vi "CRYProject Tree Action Check.vi"(8 "tag":string, 9 "Coords In":T1={"Horizontal"=-1, "Vertical"=-1}, 10 "sOption":string, 11 "Project Tree reference":refnum<vi>) -> (2 "Type Out":string, 3 "bResult":bool)   [LabVIEW 2013]
uses:
  <vilib>/Utility/miscctls.llb/LVPoint32TypeDef.ctl
  CRYProject Editor Global.vi
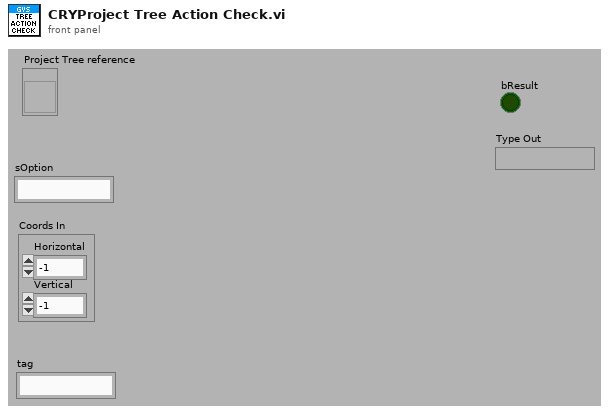
[diagram p1: front panel]
types:
  T1 = typedef "LVPoint32TypeDef.ctl" = cluster{"Horizontal":i32, "Vertical":i32}
  T2 = typedef "CRYTS.ctl" = cluster{"No.TS":u16, "TS File Path":path, "TS Name":string, "EditStepName":string, "Steps":T3[], "New State":bool, "Change State":bool, "Flattened CurveLib Data":string, "Document Data":string, "EditStepNo":u16, "Operator Start File":string, "Sequence Type":string, "Sequence Language":string}
  T3 = typedef "CRYStep.ctl" = cluster{"No.VI":i32, "Category":string, "StepName":string, "Seq setup flattened":string, "Comment":string, "Steps config.":bool[], "Jump config":i32[], "Start":dbl, "Increment":dbl, "Name":string, "Unit":string, "Y data":u16, "Y prefix":string, "Y dB ref":dbl, "Y unit":string, "Repeat State Array":cluster{"Start":dbl, "Increment":dbl, "Count":i32, "Num":i32}[]}
  T4 = enum16{"OK", "Yes", "YesNo", "YesNoCancel", "ReplaceAppend"}
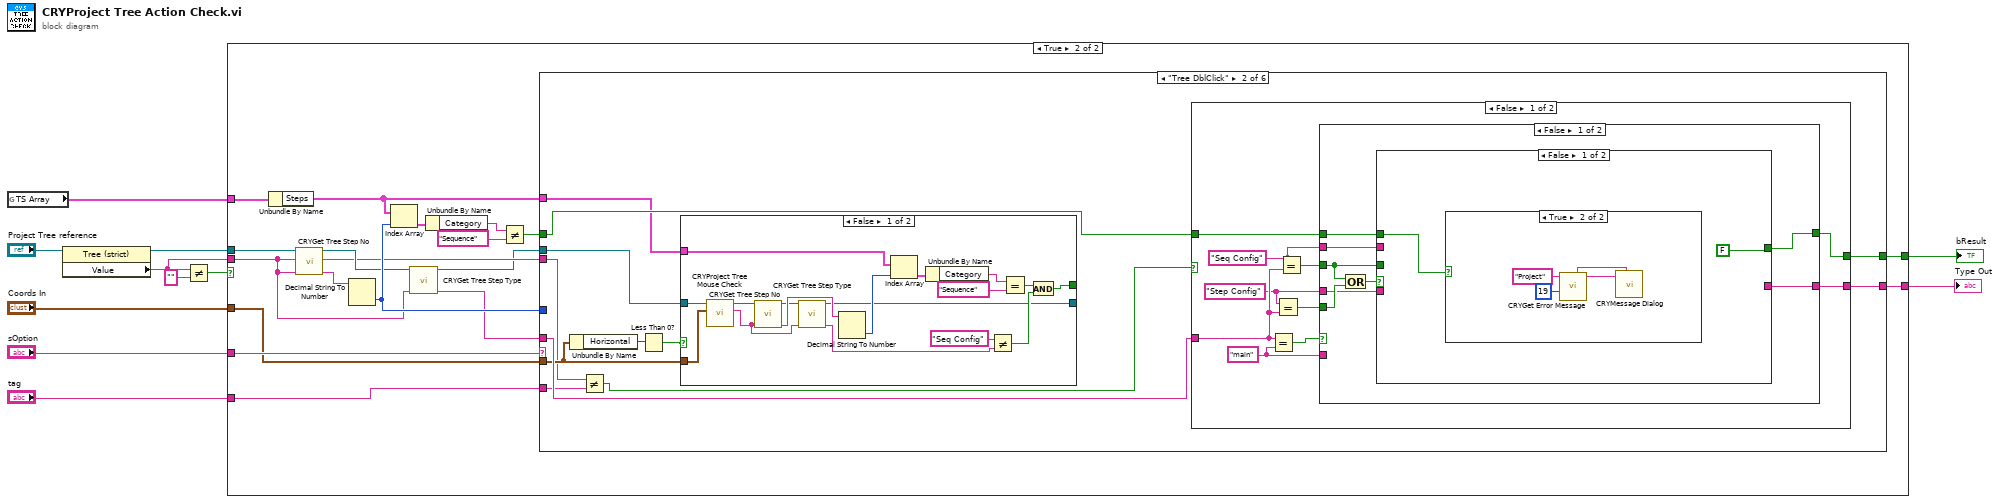
[diagram p0: block diagram]
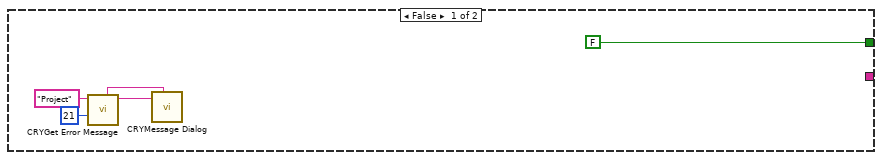
[diagram p2: hidden frame]
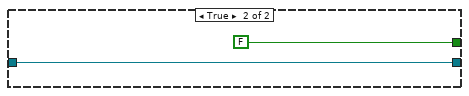
[diagram p4: hidden frame]
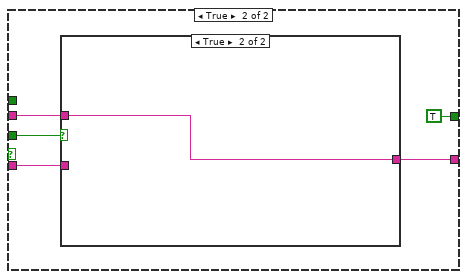
[diagram p6: hidden frame]
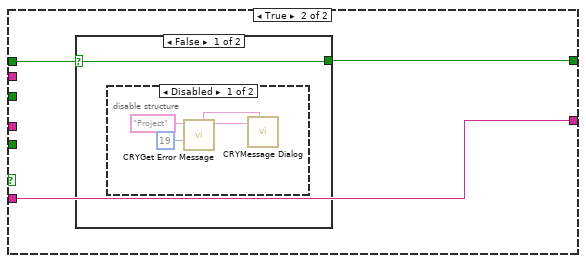
[diagram p8: hidden frame]
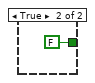
[diagram p11: hidden frame]
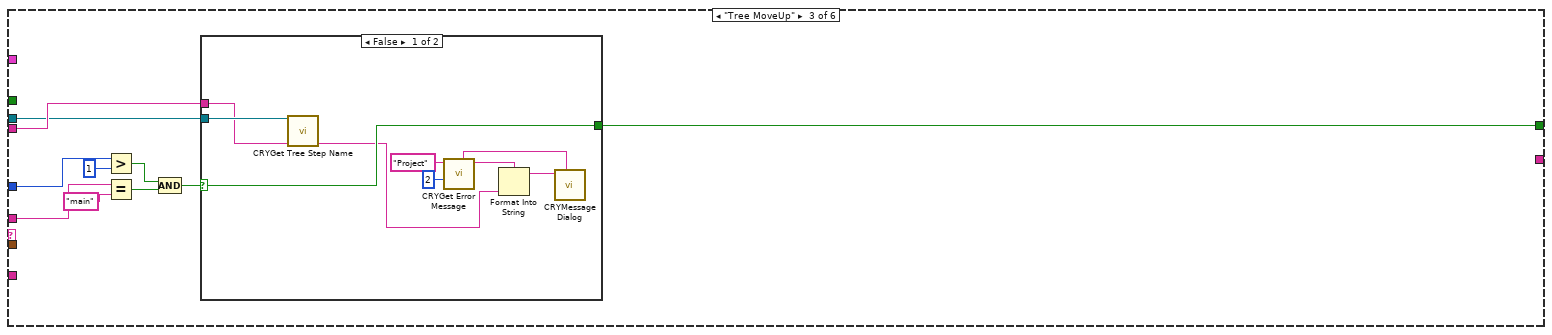
[diagram p12: hidden frame]
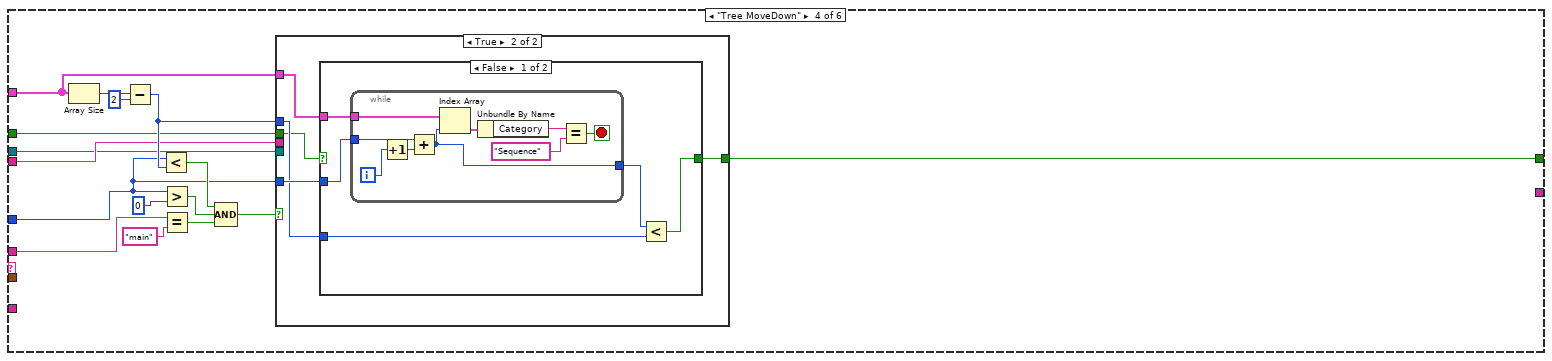
[diagram p14: hidden frame]
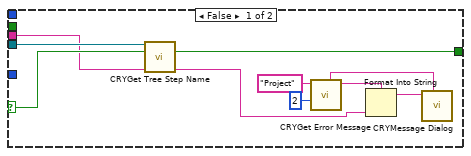
[diagram p15: hidden frame]
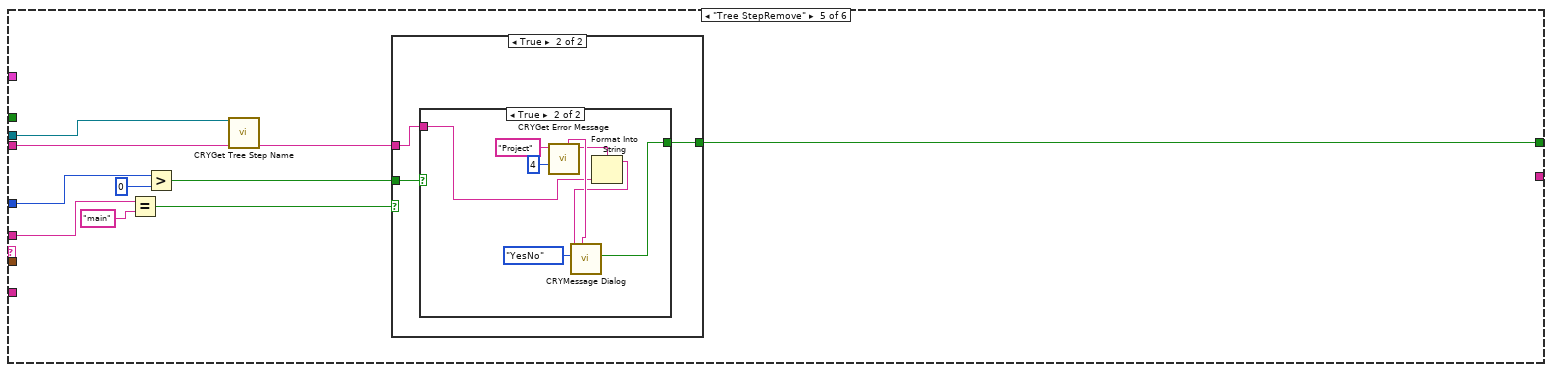
[diagram p17: hidden frame]
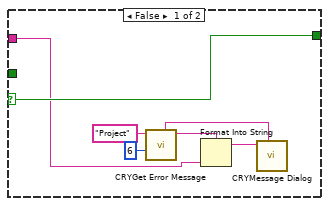
[diagram p18: hidden frame]
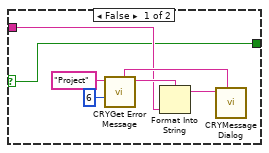
[diagram p19: hidden frame]
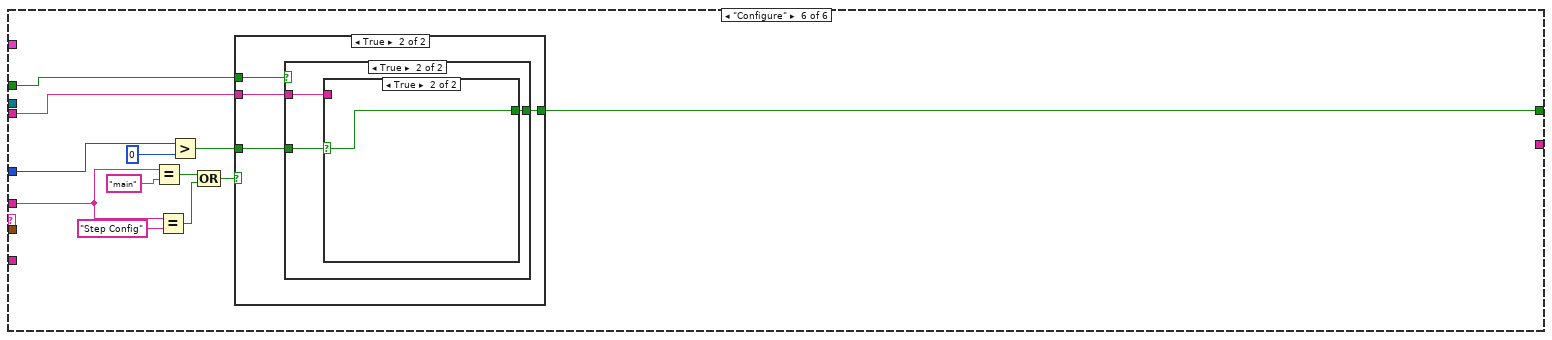
[diagram p20: hidden frame]
diagram:
  n1 = global read "CRYProject Editor Global.vi" "TS Array"() -> (w4:T2)
  n2 = property on="Property Node" class="Tree (strict)"(reference="Project Tree reference") -> (reference out=w8:refnum<vi>, "Value"=w2:string)  [unwired: 1 in, 1 out]
  n3 = Not Equal?(x=w2, y="") -> (x != y?=w7:bool)
  n4 = case shown="True" w7 {
    tunnel: [FALSE ("YesNo") w34] -> w11
    tunnel: "sOption" -> [_ w33]
    tunnel: w8 -> [_ w23]
    tunnel: w2 -> [_ w20]
    tunnel: "Coords In" -> [_ w24]
    tunnel: w4 -> [_ w31]
    tunnel: [_ w30] -> w3
    tunnel: "tag" -> [_ w17]
    frame False {
      n5 = call "CRYGet Error Message.vi"("Error No"=21, "Kind"="Project") -> ("Message"=w15:string, "Window Title"=w14:string)  [unwired: 4 in, 4 out]
      n6 = call "CRYMessage Dialog.vi"("Window Title"=w14, "Message Content"=w15) -> ()  [unwired: 8 in, 2 out]
    }
    frame True {
      n7 = Unbundle By Name(w31) -> ("Steps"=w32:T3[])
      n8 = call "CRYGet Tree Step No.vi"("SequenceTree"=w23, "Active Item Tag"=w20) -> ("reference out"=w21:refnum<vi>, "Active Cell String4"=w22:string)  [unwired: 12 in]
      n9 = Decimal String To Number(string=w22) -> (number=w25:i32)  [unwired: 2 in, 1 out]
      n10 = Index Array(array=w32, index=w25) -> (element=w28:T3)
      n11 = call "CRYGet Tree Step Type.vi"("SequenceTree"=w21, "Active Item Tag"=w20) -> ("reference out"=w18:refnum<vi>, "Active Cell String3"=w19:string)  [unwired: 12 in]
      n12 = Unbundle By Name(w28) -> ("Category"=w29:string)
      n13 = Not Equal?(x=w29, y="Sequence" ("Category")) -> (x != y?=w26:bool)
      n14 = case shown="\"Tree DblClick\"" w33 {
        tunnel: w18 -> [_ w39 w108 w129 w174 _]
        tunnel: [_ w46 w116 w142 w181 w218] -> w34
        tunnel: w32 -> [_ w38 _ w138 _ _]
        tunnel: w20 -> [_ w36 w111 w132 w173 w214]
        tunnel: w19 -> [_ w44 w110 w131 w177 w208]
        tunnel: w26 -> [_ w45 _ w128 _ w213]
        tunnel: w25 -> [_ _ w109 w130 w176 w212]
        tunnel: [_ w43 _ _ _ _] -> w30
        tunnel: w24 -> [_ w40 _ _ _ _]
        tunnel: w17 -> [_ w37 _ _ _ _]
        frame Default {
        }
        frame "Tree DblClick" {
          n15 = Unbundle By Name(w40) -> ("Horizontal"=w42:i32)
          n16 = Not Equal?(x=w36, y=w37) -> (x != y?=w35:bool)
          n17 = Less Than 0?(x=w42) -> (x < 0?=w41:bool)
          n18 = case shown="False" w41 {
            tunnel: w39 -> [w63 w65]
            tunnel: w40 -> [w62 _]
            tunnel: [w48 w65] -> _
            tunnel: w38 -> [w57 _]
            tunnel: [w55 FALSE] -> _
            frame False {
              n19 = call "CRYProject Tree Mouse Check.vi"("Coords In"=w62, "Tree Reference In"=w63) -> ("Clicked String Out"=w49:string, "Tree Reference Out"=w52:refnum<vi>)  [unwired: 8 in]
              n20 = call "CRYGet Tree Step No.vi"("SequenceTree"=w52, "Active Item Tag"=w49) -> ("reference out"=w50:refnum<vi>, "Active Cell String4"=w51:string)  [unwired: 12 in]
              n21 = call "CRYGet Tree Step Type.vi"("SequenceTree"=w50, "Active Item Tag"=w49) -> ("reference out"=w48:refnum<vi>, "Active Cell String3"=w47:string)  [unwired: 12 in]
              n22 = Decimal String To Number(string=w51) -> (number=w58:i32)  [unwired: 2 in, 1 out]
              n23 = Index Array(array=w57, index=w58) -> (element=w60:T3)
              n24 = Unbundle By Name(w60) -> ("Category"=w59:string)
              n25 = Not Equal?(x="Seq Config" ("SequenceName"), y=w47) -> (x != y?=w53:bool)
              n26 = Equal?(x=w59, y="Sequence" ("Category")) -> (x = y?=w56:bool)
              n27 = Compound Arithmetic op=AND(w56, w53) -> (w55:bool)
            }
            frame True {
            }
          }
          n28 = case shown="False" w35 {
            tunnel: [w75 FALSE] -> w46
            tunnel: w45 -> [w73 _]
            tunnel: w44 -> [w72 _]
            tunnel: [w67 _] -> w43
            frame False {
              w68 = "Step Config" ("SequenceName")
              w69 = "Seq Config" ("SequenceName")
              w66 = "main" ("decimal integer string")
              n29 = Equal?(x=w72, y=w66) -> (x = y?=w74:bool)
              n30 = Equal?(x=w68, y=w72) -> (x = y?=w70:bool)
              n31 = Equal?(x=w69, y=w72) -> (x = y?=w71:bool)
              n32 = case shown="False" w74 {
                tunnel: w73 -> [w83 w99]
                tunnel: [w79 w98] -> w75
                tunnel: w71 -> [w80 _]
                tunnel: w70 -> [w82 _]
                tunnel: w69 -> [w78 _]
                tunnel: w68 -> [w77 _]
                tunnel: [w76 w97] -> w67
                tunnel: w66 -> [_ w97]
                frame False {
                  n33 = Compound Arithmetic op=OR(w80, w82) -> (w81:bool)
                  n34 = case shown="False" w81 {
                    tunnel: w83 -> [w85 _]
                    tunnel: w80 -> [_ w94]
                    tunnel: [FALSE TRUE] -> w79
                    tunnel: w78 -> [_ w92]
                    tunnel: w77 -> [_ w91]
                    tunnel: [_ w90] -> w76
                    frame False {
                      n35 = case shown="True" w85 {
                        frame False {
                        }
                        frame True {
                          n36 = call "CRYGet Error Message.vi"("Error No"=19, "Kind"="Project") -> ("Message"=w89:string, "Window Title"=w88:string)  [unwired: 4 in, 4 out]
                          n37 = call "CRYMessage Dialog.vi"("Window Title"=w88, "Message Content"=w89) -> ()  [unwired: 8 in, 2 out]
                        }
                      }
                    }
                    frame True {
                      n38 = case shown="True" w94 {
                        tunnel: w92 -> [_ w96]
                        tunnel: w91 -> [w95 _]
                        tunnel: [w95 w96] -> w90
                        frame False {
                        }
                        frame True {
                        }
                      }
                    }
                  }
                }
                frame True {
                  n39 = case shown="False" w99 {
                    selector: w99 -> [w100 w105]
                    tunnel: [w100 w105] -> w98
                    frame False {
                      n40 = disable-structure shown="Disabled" {
                        frame Disabled {
                          n41 = call "CRYGet Error Message.vi"("Error No"=19, "Kind"="Project") -> ("Message"=w104:string, "Window Title"=w103:string)  [unwired: 4 in, 4 out]
                          n42 = call "CRYMessage Dialog.vi"("Window Title"=w103, "Message Content"=w104) -> ()  [unwired: 8 in, 2 out]
                        }
                        frame Enabled {
                        }
                      }
                    }
                    frame True {
                    }
                  }
                }
              }
            }
            frame True {
            }
          }
        }
        frame "Tree MoveUp" {
          n43 = Greater?(x=w109, y=1) -> (0:w112:bool)
          n44 = Equal?(x=w110, y="main" ("decimal integer string")) -> (x = y?=w115:bool)
          n45 = Compound Arithmetic op=AND(w112, w115) -> (w114:bool)
          n46 = case shown="False" w114 {
            selector: w114 -> [w120 w126]
            tunnel: [w120 w126] -> w116
            tunnel: w108 -> [w119 _]
            tunnel: w111 -> [w118 _]
            frame False {
              n47 = call "CRYGet Tree Step Name.vi"("SequenceTree"=w119, "Active Item Tag"=w118) -> ("Active Cell String0"=w117:string)  [unwired: 12 in, 1 out]
              n48 = call "CRYGet Error Message.vi"("Error No"=2, "Kind"="Project") -> ("Message"=w123:string, "Window Title"=w125:string)  [unwired: 4 in, 4 out]
              n49 = Format Into String(format string=w123, w117) -> (resulting string=w124:string)  [unwired: 2 in, 1 out]
              n50 = call "CRYMessage Dialog.vi"("Window Title"=w125, "Message Content"=w124) -> ()  [unwired: 8 in, 2 out]
            }
            frame True {
            }
          }
        }
        frame "Tree MoveDown" {
          n51 = Array Size(array=w138) -> (size(s)=w141:i32)
          n52 = Subtract(x=w141, y=2) -> (x-y=w139:i32)
          n53 = Less?(x=w130, y=w139) -> (x < y?=w133:bool)
          n54 = Greater?(x=w130, y=0) -> (0:w135:bool)
          n55 = Equal?(x=w131, y="main" ("decimal integer string")) -> (x = y?=w137:bool)
          n56 = Compound Arithmetic op=AND(w133, w135, w137) -> (w136:bool)
          n57 = case shown="True" w136 {
            selector: w136 -> [w146 _]
            tunnel: [w146 w156] -> w142
            tunnel: w132 -> [w144 _]
            tunnel: w138 -> [_ w155]
            tunnel: w130 -> [_ w154]
            tunnel: w139 -> [_ w153]
            tunnel: w129 -> [w145 _]
            tunnel: w128 -> [_ w152]
            frame False {
              n58 = call "CRYGet Tree Step Name.vi"("SequenceTree"=w145, "Active Item Tag"=w144) -> ("Active Cell String0"=w143:string)  [unwired: 12 in, 1 out]
              n59 = call "CRYGet Error Message.vi"("Error No"=2, "Kind"="Project") -> ("Message"=w149:string, "Window Title"=w151:string)  [unwired: 4 in, 4 out]
              n60 = Format Into String(format string=w149, w143) -> (resulting string=w150:string)  [unwired: 2 in, 1 out]
              n61 = call "CRYMessage Dialog.vi"("Window Title"=w151, "Message Content"=w150) -> ()  [unwired: 8 in, 2 out]
            }
            frame True {
              n62 = case shown="False" w152 {
                selector: w152 -> [_ w171]
                tunnel: [w157 w171] -> w156
                tunnel: w155 -> [w161 _]
                tunnel: w154 -> [w160 _]
                tunnel: w153 -> [w158 _]
                frame False {
                  n63 = while {
                    tunnel: w161 -> [w170]
                    tunnel: w160 -> [w169]
                    tunnel: [w162] -> w159
                    i -> [w163]
                    stop <- w164 stop-if-true
                    n64 = Increment(x=w163) -> (x+1=w168:i32)
                    n65 = Add(x=w169, y=w168) -> (x+y=w162:i32)
                    n66 = Index Array(array=w170, index=w162) -> (element=w167:T3)
                    n67 = Unbundle By Name(w167) -> ("Category"=w166:string)
                    n68 = Equal?(x=w166, y="Sequence") -> (x = y?=w164:bool)
                  }
                  n69 = Less?(x=w159, y=w158) -> (x < y?=w157:bool)
                }
                frame True {
                }
              }
            }
          }
        }
        frame "Tree StepRemove" {
          n70 = Equal?(x=w177, y="main" ("decimal integer string")) -> (x = y?=w180:bool)
          n71 = Greater?(x=w176, y=0) -> (0:w178:bool)
          n72 = call "CRYGet Tree Step Name.vi"("SequenceTree"=w174, "Active Item Tag"=w173) -> ("Active Cell String0"=w172:string)  [unwired: 12 in, 1 out]
          n73 = case shown="True" w180 {
            selector: w180 -> [w188 _]
            tunnel: [w188 w191] -> w181
            tunnel: w172 -> [w182 w190]
            tunnel: w178 -> [_ w189]
            frame False {
              n74 = call "CRYGet Error Message.vi"("Error No"=6, "Kind"="Project") -> ("Message"=w185:string, "Window Title"=w187:string)  [unwired: 4 in, 4 out]
              n75 = Format Into String(format string=w185, w182) -> (resulting string=w186:string)  [unwired: 2 in, 1 out]
              n76 = call "CRYMessage Dialog.vi"("Window Title"=w187, "Message Content"=w186) -> ()  [unwired: 8 in, 2 out]
            }
            frame True {
              n77 = case shown="True" w189 {
                selector: w189 -> [w192 _]
                tunnel: [w192 w200] -> w191
                tunnel: w190 -> [w193 w199]
                frame False {
                  n78 = call "CRYGet Error Message.vi"("Error No"=6, "Kind"="Project") -> ("Message"=w196:string, "Window Title"=w198:string)  [unwired: 4 in, 4 out]
                  n79 = Format Into String(format string=w196, w193) -> (resulting string=w197:string)  [unwired: 2 in, 1 out]
                  n80 = call "CRYMessage Dialog.vi"("Window Title"=w198, "Message Content"=w197) -> ()  [unwired: 8 in, 2 out]
                }
                frame True {
                  n81 = call "CRYGet Error Message.vi"("Error No"=4, "Kind"="Project") -> ("Message"=w203:string, "Window Title"=w205:string)  [unwired: 4 in, 4 out]
                  n82 = Format Into String(format string=w203, w199) -> (resulting string=w204:string)  [unwired: 2 in, 1 out]
                  n83 = call "CRYMessage Dialog.vi"("Window Title"=w205, "YesNoCancel"=T4."YesNo", "Message Content"=w204) -> ("YesNo"=w200:bool)  [unwired: 7 in, 1 out]
                }
              }
            }
          }
        }
        frame "Configure" {
          n84 = Equal?(x=w208, y="main" ("decimal integer string")) -> (x = y?=w217:bool)
          n85 = Equal?(x=w208, y="Step Config" ("SequenceName")) -> (x = y?=w209:bool)
          n86 = Greater?(x=w212, y=0) -> (0:w215:bool)
          n87 = Compound Arithmetic op=OR(w217, w209) -> (w210:bool)
          n88 = case shown="True" w210 {
            selector: w210 -> [w224 _]
            tunnel: [w224 w228] -> w218
            tunnel: w214 -> [_ w227]
            tunnel: w215 -> [_ w226]
            tunnel: w213 -> [_ w225]
            frame False {
              n89 = call "CRYGet Error Message.vi"("Error No"=18, "Kind"="Project") -> ("Message"=w223:string, "Window Title"=w219:string)  [unwired: 4 in, 4 out]
              n90 = call "CRYMessage Dialog.vi"("Window Title"=w219, "YesNoCancel"=T4."OK", "Message Content"=w223) -> ()  [unwired: 7 in, 2 out]
            }
            frame True {
              n91 = case shown="True" w225 {
                selector: w225 -> [w234 _]
                tunnel: [w234 w237] -> w228
                tunnel: w227 -> [_ w236]
                tunnel: w226 -> [_ w235]
                frame False {
                  n92 = call "CRYGet Error Message.vi"("Error No"=18, "Kind"="Project") -> ("Message"=w233:string, "Window Title"=w229:string)  [unwired: 4 in, 4 out]
                  n93 = call "CRYMessage Dialog.vi"("Window Title"=w229, "YesNoCancel"=T4."OK", "Message Content"=w233) -> ()  [unwired: 7 in, 2 out]
                }
                frame True {
                  n94 = case shown="True" w235 {
                    selector: w235 -> [w243 w244]
                    tunnel: [w243 w244] -> w237
                    tunnel: w236 -> [_ _]
                    frame False {
                      n95 = call "CRYGet Error Message.vi"("Error No"=1, "Kind"="Project") -> ("Message"=w240:string, "Window Title"=w241:string)  [unwired: 4 in, 4 out]
                      n96 = call "CRYMessage Dialog.vi"("Window Title"=w241, "YesNoCancel"=T4."OK", "Message Content"=w240) -> ()  [unwired: 7 in, 2 out]
                    }
                    frame True {
                    }
                  }
                }
              }
            }
          }
        }
      }
    }
  }
  "bResult" <- w11
  "Type Out" <- w3
